vi "PV filter.vi"(1 "iteration":i32, 2 "process variable":dbl format="%.2f") -> (0 "filtered pv":dbl format="%.2f")   [LabVIEW 2020, in "NI_PID__prctrl compat.lvlib"]
doc: "This VI implements a simple filter on the measured process variable. The VI may be removed if filtering is not necessary or modified if additional filtering is needed to remove measured noise on the process variable."
uses:
  <vilib>/addons/control/pid/NI_PID__prctrl compat.lvlib
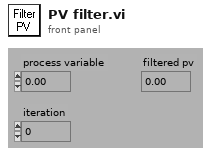
[diagram p1: front panel]
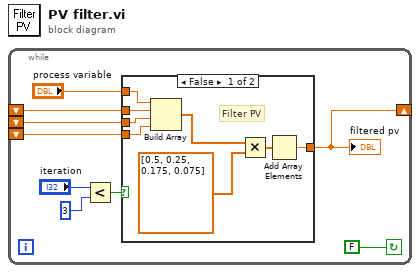
[diagram p0: block diagram]
diagram:
  n1 = while {
    shift-left: _ -> [w3]
    shift-left: _ -> [w2]
    shift-left: _ -> [w5]
    shift-right: [w4] -> _
    stop <- FALSE continue-if-true
    n2 = Less?(x="iteration", y=3) -> (x < y?=w9:bool)
    n3 = case shown="False" w9 {
      tunnel: w3 -> [w11 _]
      tunnel: w2 -> [w12 _]
      tunnel: w5 -> [w13 _]
      tunnel: "process variable" -> [w17 w18]
      tunnel: [w14 w18] -> w4
      frame False {
        # "Filter PV"
        n4 = Build Array(w17, w13, w12, w11) -> (w16:dbl[])
        n5 = Multiply(x=w16, y=dbl[] [0.5, 0.25, 0.175, 0.075]) -> (x*y=w15:dbl[])
        n6 = Add Array Elements(numeric array=w15) -> (sum=w14:dbl)
      }
      frame True {
        # "Do not filter PV"
      }
    }
    "filtered pv" <- w4
  }
